vi "Duplicate Disabled Frame.vi"(8 "Error In":errorcluster, 11 "DisableStructure In":refnum<vi>) -> (0 "Error Out":errorcluster, 3 "DisableStructure Out":refnum<vi>)   [LabVIEW 2017, in "Toolkit.lvlib"]
uses:
  Toolkit.lvlib
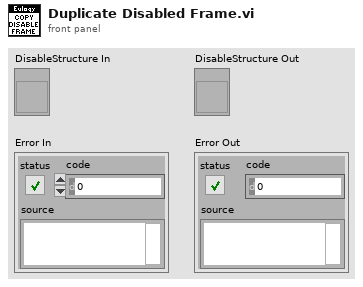
[diagram p1: front panel]
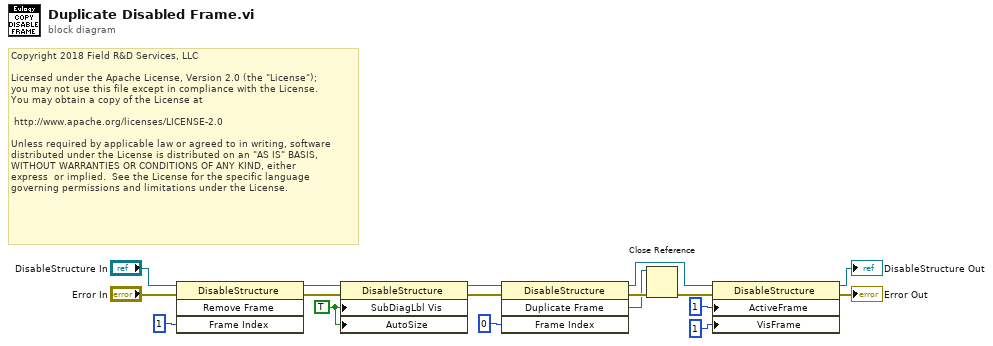
[diagram p0: block diagram]
diagram:
  w13 = TRUE ("Subdiagram Label Visible")
  # "Copyright 2018 Field R&D Services, LLC\n\nLicensed under the Apache License, Version 2.0 (the \"License\");\nyou may not use this file except in compliance with the License.\nYou may obtain a copy of the License at\n\n\thttp://www.apache.org/licenses/LICENSE-2.0\n\nUnless required by applicable law or agreed to in writing, software\ndistributed under the License is distributed on an \"AS IS\" BASIS,\nWITHOUT WARRANTIES OR CONDITIONS OF ANY KIND, either \nexpress  or implied.  See the License for the specific language \ngoverning permissions and limitations under the License."
  n1 = invoke class="DisableStructure" method="Remove Frame"(reference="DisableStructure In", error in="Error In", "Frame Index"=u32 1) -> (reference out=w3:refnum<vi>, error out=w9:errorcluster)  [unwired: 1 in, 2 out]
  n2 = property class="DisableStructure"(reference=w3, error in=w9, "SubDiagLbl Vis"=w13, "AutoSize"=w13) -> (reference out=w8:refnum<vi>, error out=w10:errorcluster)
  n3 = invoke class="DisableStructure" method="Duplicate Frame"(reference=w8, error in=w10, "Frame Index"=u32 0) -> (reference out=w7:refnum<vi>, error out=w5:errorcluster, "Duplicate Frame"=w1:refnum<vi>)  [unwired: 1 in, 1 out]
  n4 = Close Reference(reference=w1, error in (no error)=w5) -> (error out=w2:errorcluster)
  n5 = property class="DisableStructure"(reference=w7, error in=w2, "ActiveFrame"=i16 1 ("Active Frame"), "VisFrame"=u32 1 ("Visible Frame")) -> (reference out=→"DisableStructure Out":refnum<vi>, error out=→"Error Out":errorcluster)
